vi "Classification Particle Analysis.vi"(8 "error in (no error)":errorcluster, 10 "Image Dest":T1, 11 "Image Source":T1) -> (0 "error out":errorcluster, 1 "Center of Masses":cluster{"X":dbl, "Y":dbl}[](array[cluster]), 2 "ROIs":T2[](array[typedef]) {"Contours"."Type" items=["No Selection", "Point", "Line", "Rectangle", "Oval", "Polygon", "Freehand Region", "Annulus", "Unused2", "Unused3", "Broken Line", "Freehand Line", "Rotated Rectangle"]}, 3 "Image Out":T1)   [LabVIEW 2017]
doc: "This VI helps filter out unwanted particles and returns bounding box and center of mass information for the remaining particles."
uses:
  <vilib>/vision/Image Controls.llb/IMAQ Image.ctl
  <vilib>/vision/NI_Vision_Development_Module.lvlib
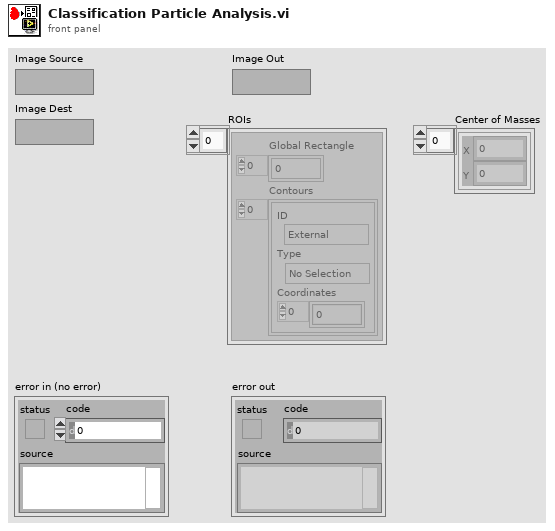
[diagram p1: front panel]
types:
  T1 = typedef "IMAQ Image.ctl" = refnum<image>
  T2 = typedef "ROI Descriptor" = cluster{"Global Rectangle":i32[], "Contours":cluster{"ID":enum32{"External", "Internal"}, "Type":u32, "Coordinates":i32[]}[]}
  T3 = cluster{"Area":dbl, "Number of Holes":dbl, "Bounding Rect":cluster{"Left":dbl, "Top":dbl, "Right":dbl, "Bottom":dbl}, "Center of Mass":cluster{"X":dbl, "Y":dbl}, "Orientation":dbl, "Dimensions":cluster{"Width":dbl, "Height":dbl}}[]
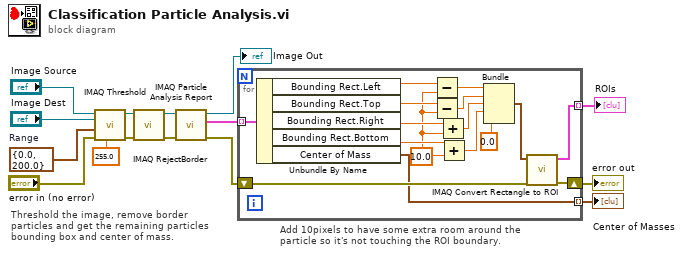
[diagram p0: block diagram]
diagram:
  w15 = cluster{"Lower value":sgl, "Upper value":sgl} {"Lower value"=0.0, "Upper value"=200.0}  # Range
  # "Add 10pixels to have some extra room around the particle so it's not touching the ROI boundary."
  # "Threshold the image, remove border particles and get the remaining particles bounding box and center of mass."
  n1 = call "IMAQ Threshold"("Replace Value"=sgl 255.0, "error in (no error)"="error in (no error)", "Range"=w15, "Image Dst"="Image Dest", "Image Src"="Image Source") -> ("error out"=w4:errorcluster, "Image Dst Out"=w5:T1)  [unwired: 1 in, 4 out]
  n2 = call "IMAQ RejectBorder"("error in (no error)"=w4, "Image Src"=w5) -> ("error out"=w2:errorcluster, "Image Dst Out"=w3:T1)  [unwired: 2 in, 2 out]
  n3 = call "IMAQ Particle Analysis Report"("error in (no error)"=w2, "Image"=w3) -> ("error out"=w11:errorcluster, "Particle Reports (Pixels)"=w13:T3, "Image Out (duplicate)"=→"Image Out":T1)  [unwired: 1 in, 6 out]
  n4 = for {
    tunnel: w13 -> [w31] mode=indexing
    tunnel: [w29] -> w12 mode=indexing
    shift-right: [w27] -> w10
    shift-left: w11 -> [w28]
    tunnel: [w26] -> w9 mode=indexing
    w18 = 10.0
    n5 = Unbundle By Name(w31) -> ("Bounding Rect.Left"=w25:dbl, "Bounding Rect.Top"=w24:dbl, "Bounding Rect.Right"=w21:dbl, "Bounding Rect.Bottom"=w20:dbl, "Center of Mass"=w26:cluster{"X":dbl, "Y":dbl})
    n6 = Subtract(x=w25, y=w18) -> (x-y=w23:dbl)
    n7 = Subtract(x=w24, y=w18) -> (x-y=w22:dbl)
    n8 = Add(x=w21, y=w18) -> (x+y=w16:dbl)
    n9 = Add(x=w20, y=w18) -> (x+y=w19:dbl)
    n10 = Bundle(w23, w22, w16, w19, 0.0) -> (w17:cluster{dbl, dbl, dbl, dbl, dbl})  [unwired: 1 out]
    n11 = call "IMAQ Convert Rectangle to ROI"("error in (no error)"=w28, "Rectangle"=w17) -> ("error out"=w27:errorcluster, "ROI Descriptor"=w29:T2)  [unwired: 7 out]
  }
  "ROIs" <- w12
  "error out" <- w10
  "Center of Masses" <- w9
